vi "Get Actual Temperature.vi"(8 "error in (no error)":errorcluster, 10 "Time Stamp":timestamp, 11 "Thermal Chamber Response Simlator In":refnum<class "Thermal Chamber Response Simlator.lvclass">) -> (0 "error out":errorcluster, 2 "Actual Temperature [degC]":dbl, 3 "Thermal Chamber Response Simlator Out":refnum<class "Thermal Chamber Response Simlator.lvclass">)   [LabVIEW 2020, in "Thermal Chamber Response Simlator.lvclass"]
uses:
  Thermal Chamber Response Simlator.lvclass
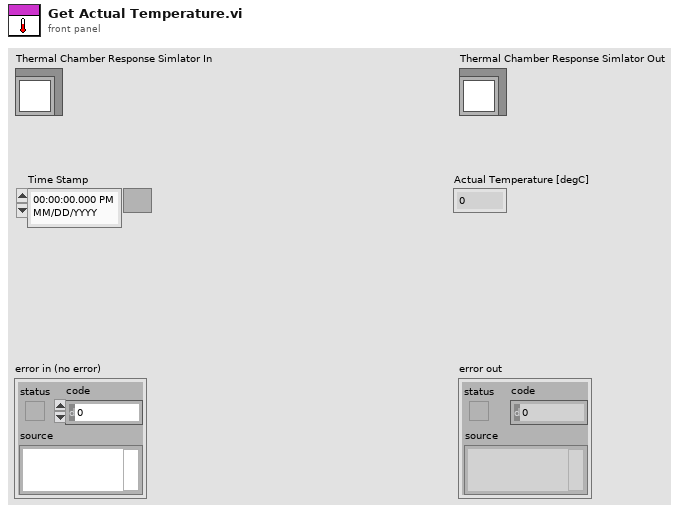
[diagram p1: front panel]
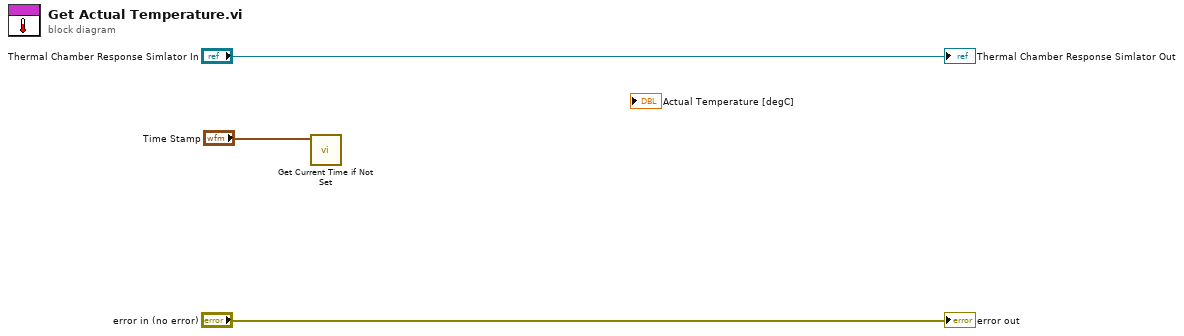
[diagram p0: block diagram]
diagram:
  n1 = call "Get Current Time if Not Set.vi"("Start Time"="Time Stamp") -> ()  [unwired: 10 in, 1 out]
  "error out" <- "error in (no error)"
  "Thermal Chamber Response Simlator Out" <- "Thermal Chamber Response Simlator In"
